vi "GetBindings.vi"(8 "error in (no error)":errorcluster) -> (0 "error out":errorcluster, 3 "Binding Info":T1)   [LabVIEW 2014, in "Template SoftMotion Drive Interface Plug-in Class.lvclass"]
uses:
  Template SoftMotion Drive Interface Plug-in Class.lvclass
  <vilib>/Motion/plugins/PluginFramework/nismSDIFramework.Binding.ctl
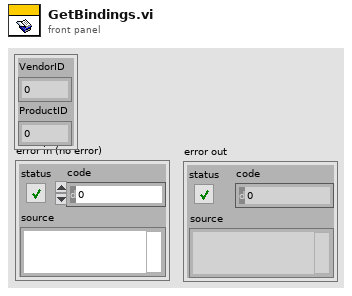
[diagram p1: front panel]
types:
  T1 = typedef "nismSDIFramework.Binding.ctl" = cluster{"VendorID":u32, "ProductID":u32}
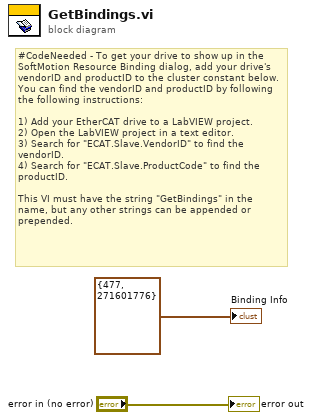
[diagram p0: block diagram]
diagram:
  # "#CodeNeeded - To get your drive to show up in the SoftMotion Resource Binding dialog, add your drive's vendorID and productID to the cluster constant below. You can find the vendorID and productID by following the following instructions:\n\n1) Add your EtherCAT drive to a LabVIEW project.\n2) Open the LabVIEW project in a text editor.\n3) Search for \"ECAT.Slave.VendorID\" to find the vendorID.\n4) Search for \"ECAT.Slave.ProductCode\" to find the productID. \n\nThis VI must have the string \"GetBindings\" in the name, but any other strings can be appended or prepended."
  "error out" <- "error in (no error)"
  "Binding Info" <- T1 {"VendorID"=477, "ProductID"=271601776} ("Binding Info")
